vi "Get Data.vi"(8 "error in (no error)":errorcluster, 11 "DataGrid.lvlib:Abstract EVENT.lvclass":refnum<class "Abstract EVENT.lvclass">) -> (0 "error out":errorcluster, 1 "column":i32, 2 "row":i32)   [LabVIEW 2013, in "DataGrid.lvlib" / "CellClick.lvclass"]
doc: "Converts the class data for cell click into individual components of the grid"
uses:
  CellClick.lvclass
  Abstract EVENT/Abstract EVENT.lvclass
  CellClick.lvclass/CellClick.ctl
  Read column.vi
  Read row.vi
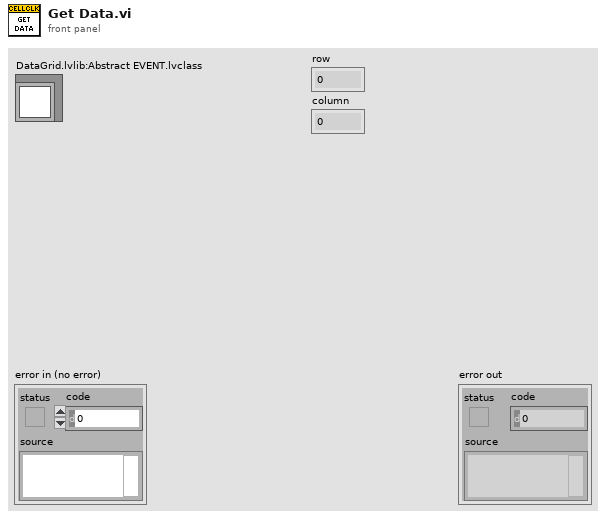
[diagram p1: front panel]
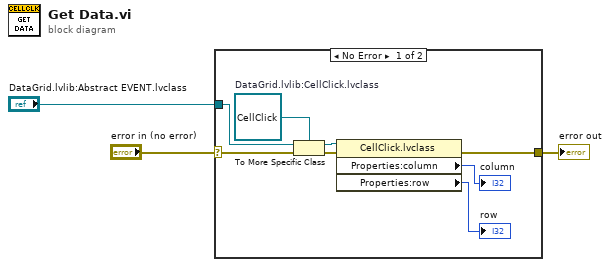
[diagram p0: block diagram]
diagram:
  n1 = case shown="No Error" "error in (no error)" {
    selector: "error in (no error)" -> [w8 w12]
    tunnel: [w7 w12] -> w2
    tunnel: "DataGrid.lvlib:Abstract EVENT.lvclass" -> [w9 _]
    frame No Error {
      w6 = refnum<class "CellClick.lvclass"> refnum  # DataGrid.lvlib:CellClick.lvclass
      n2 = To More Specific Class(target class=w6, reference=w9, error in=w8) -> (specific class reference=w11:refnum<class "CellClick.lvclass">, error out=w10:errorcluster)
      n3 = property class="CellClick.lvclass"(reference=w11, error in=w10) -> (error out=w7:errorcluster, "Properties:column"=→"column":i32, "Properties:row"=→"row":i32)  [unwired: 1 out]
    }
    frame Error {
    }
  }
  "error out" <- w2
